vi "SSIM.vi"() -> ()   [LabVIEW 2014]
doc: "This example shows how to use the Structural Similarity Analysis tools in NI Vision. \n\nSSIM is a metric used to determine the Similarity of an Image with respect to a Reference Image. The Reference Image is assumed to be of perfect quality. SSIM uses a window based approach and uses the structural information to determine the similarity unlike the Mean Square Error which isolates the pixels from its neighbouring pixels.\n\nThere are two SSIM techniques. Fast and Normal SSIM. Fast SSIM uses faster approaches to calculate the mean and variance. Fast SSIM calculates mean by averaging pixel values in the local window whereas Normal SSIM uses a Gaussian weighting function."
uses:
  <vilib>/vision/NI_Vision_Development_Module.lvlib
panel:
  in  "Reference Image File Path":path
  in  "Window Size":i32=8 min=3 max=65
  out "MSE Map":T1(plugin-control)
  out "Mean Square Error":dbl
  in  "Test Image File Path":path
  out "Mean SSIM*":dbl
  in  "Fast/Normal":bool=TRUE
  out "SSIM Map":T1(plugin-control)
  out "Test Image":T1(plugin-control)
  out "Reference Image":T1(plugin-control)
  in  "Stop":bool
  # "Overview: Demonstrates how to compare two image using SSIM algorithm.\nRequirements: NI Vision Development Module\nInstructions:\n1. Run the VI\n2. Select different images using the Test Image File Path control\n3. Compare the SSIM similarity metric result to a simple mean square error computation."
  # "Comparison Results"
  # "SSIM Options"
  # "* In SSIM the value 1 indicates the images are similar, the value 0 indicates the images are dissimilar."
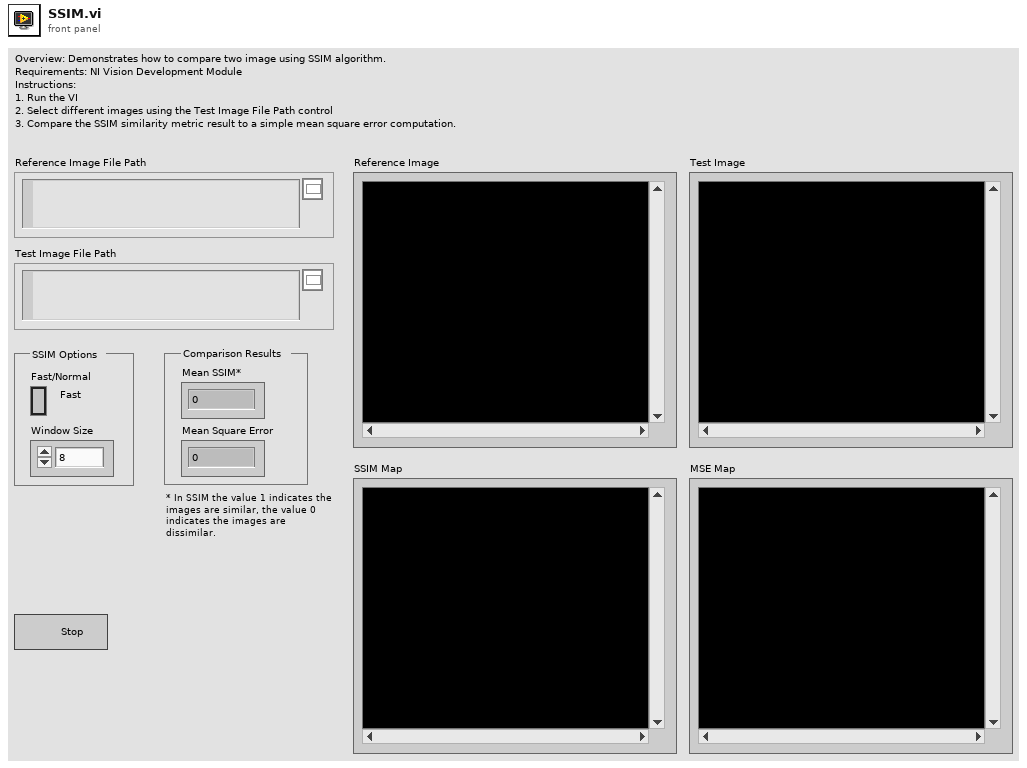
[diagram p1: front panel]
types:
  T1 = typedef "IMAQ Image.ctl" = refnum<image>
  T2 = typedef "Image Type" = u32
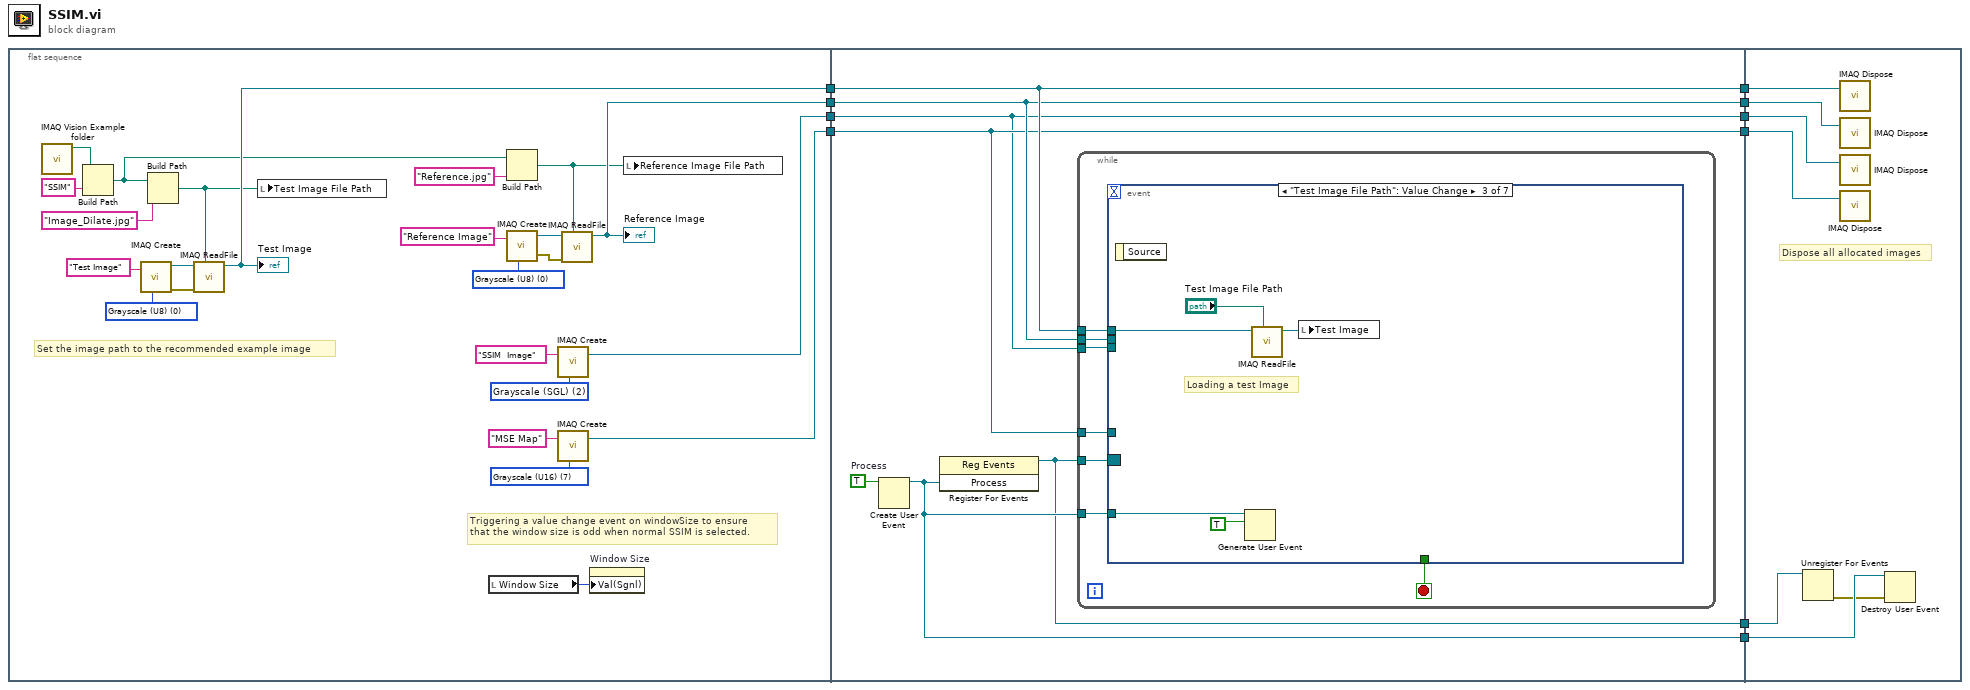
[diagram p0: block diagram]
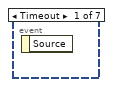
[diagram p2: hidden frame]
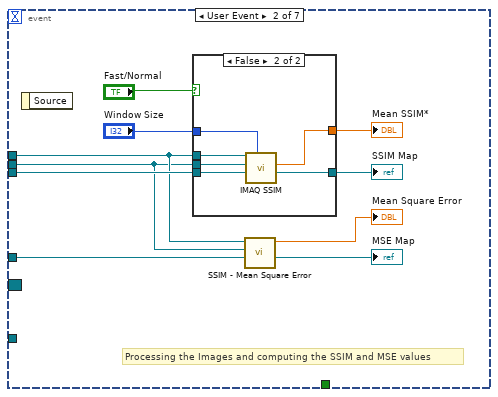
[diagram p3: hidden frame]
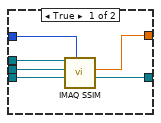
[diagram p4: hidden frame]
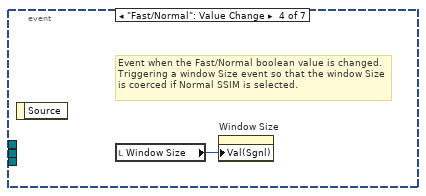
[diagram p5: hidden frame]
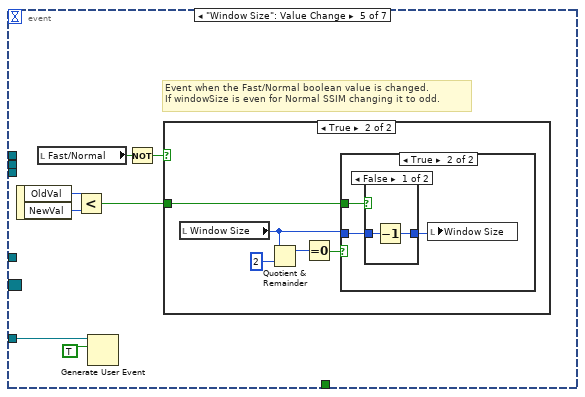
[diagram p6: hidden frame]
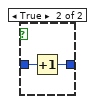
[diagram p9: hidden frame]
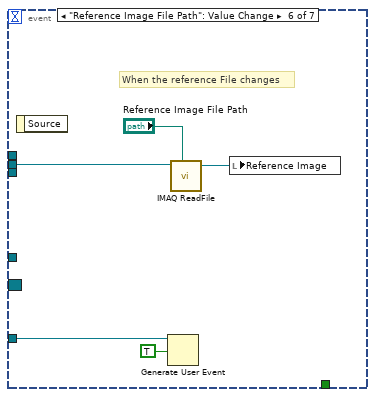
[diagram p10: hidden frame]
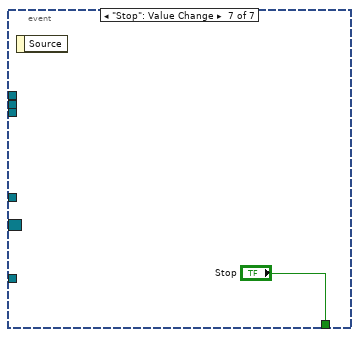
[diagram p11: hidden frame]
diagram:
  n1 = flat-sequence {
    tunnel: [w15] -> w10
    tunnel: [w14] -> w9
    tunnel: [w23] -> w8
    tunnel: [w20] -> w7
    tunnel: w10 -> [w41]
    tunnel: [w41] -> w6
    tunnel: w9 -> [w35]
    tunnel: [w35] -> w5
    tunnel: w8 -> [w40]
    tunnel: [w40] -> w4
    tunnel: w7 -> [w38]
    tunnel: [w38] -> w3
    tunnel: [w37] -> w2
    tunnel: [w36] -> w1
    tunnel: w6 -> [w108]
    tunnel: w5 -> [w104]
    tunnel: w4 -> [w102]
    tunnel: w3 -> [w107]
    tunnel: w2 -> [w105]
    tunnel: w1 -> [w106]
    frame #0 {
      w21 = T2 7 items=["Grayscale (U8)", "Grayscale (I16)", "Grayscale (SGL)", "Complex (CSG)", "RGB (U32)", "HSL (U32)", "RGB (U64)", "Grayscale (U16)"] ("Image Type")
      w25 = T2 2 items=["Grayscale (U8)", "Grayscale (I16)", "Grayscale (SGL)", "Complex (CSG)", "RGB (U32)", "HSL (U32)", "RGB (U64)"] ("Image Type")
      w31 = T2 0 items=["Grayscale (U8)", "Grayscale (I16)", "Grayscale (SGL)", "Complex (CSG)", "RGB (U32)", "HSL (U32)", "RGB (U64)"] ("Image Type")
      w32 = T2 0 items=["Grayscale (U8)", "Grayscale (I16)", "Grayscale (SGL)", "Complex (CSG)", "RGB (U32)", "HSL (U32)", "RGB (U64)"] ("Image Type")
      # "Triggering a value change event on windowSize to ensure \nthat the window size is odd when normal SSIM is selected."
      # "Set the image path to the recommended example image"
      n2 = call "IMAQ Vision Example folder.vi"() -> ("Example Image Path"=w27:path)  [unwired: 11 in]
      n3 = Build Path(base path=w27, name or relative path="SSIM") -> (appended path=w11:path)
      n4 = call "IMAQ Create"("Image Name"="Test Image", "Image Type"=w32) -> ("New Image"=w18:T1, "error out"=w17:errorcluster)  [unwired: 2 in, 1 out]
      n5 = Build Path(base path=w11, name or relative path="Image_Dilate.jpg") -> (appended path=w12:path)
      n6 = call "IMAQ ReadFile"("File Path"=w12, "error in (no error)"=w17, "Image"=w18) -> ("Image Out"=w15:T1)  [unwired: 2 in, 6 out]
      "Test Image" <- w15
      n7 = local write "Test Image File Path"(w12) -> ()
      n8 = local read "Window Size"() -> (w19:i32)
      n9 = Build Path(base path=w11, name or relative path="Reference.jpg") -> (appended path=w13:path)
      n10 = call "IMAQ Create"("Image Name"="Reference Image", "Image Type"=w31) -> ("New Image"=w30:T1, "error out"=w29:errorcluster)  [unwired: 2 in, 1 out]
      n11 = call "IMAQ Create"("Image Name"="SSIM  Image", "Image Type"=w25) -> ("New Image"=w14:T1)  [unwired: 2 in, 2 out]
      n12 = call "IMAQ Create"("Image Name"="MSE Map", "Image Type"=w21) -> ("New Image"=w20:T1)  [unwired: 2 in, 2 out]
      n13 = call "IMAQ ReadFile"("File Path"=w13, "error in (no error)"=w29, "Image"=w30) -> ("Image Out"=w23:T1)  [unwired: 2 in, 6 out]
      "Reference Image" <- w23
      n14 = property on="Window Size" class="DigNum (strict)"("Val(Sgnl)"=w19) -> ()  [unwired: 2 in, 2 out]
      n15 = local write "Reference Image File Path"(w13) -> ()
    }
    frame #1 {
      w39 = TRUE  # Process
      n16 = Create User Event(user event datatype=w39) -> (user event=w37:refnum<user-event>)  [unwired: 1 in, 1 out]
      n17 = register-events(w37) -> (reference out=w36:refnum<event-registration>)  [unwired: 2 in, 1 out]
      n18 = while {
        tunnel: w41 -> [w48]
        tunnel: w35 -> [w47]
        tunnel: w40 -> [w46]
        tunnel: w38 -> [w45]
        tunnel: w37 -> [w44]
        tunnel: w36 -> [w42]
        stop <- w43 stop-if-true
        n19 = event shown="[2] \"Test Image File Path\": Value Change" {
          selector: w42 -> [_ _ _ _ _ _ _]
          dyn-events: _ -> [_ _ _ _ _ _ _]
          timeout: _ -> [_ _ _ _ _ _ _]
          tunnel: w48 -> [_ w53 w75 _ _ _ _]
          tunnel: w47 -> [_ w58 _ _ _ _ _]
          tunnel: w46 -> [_ w52 _ _ _ w100 _]
          tunnel: w45 -> [_ w51 _ _ _ _ _]
          tunnel: w44 -> [_ _ w73 _ w83 w96 _]
          tunnel: [_ _ _ _ _ _ "Stop"] -> w43
          event Timeout {
            n20 = event-data() -> ()  [unwired: 2 out]
          }
          event User Event {
            # "Processing the Images and computing the SSIM and MSE values"
            n21 = event-data() -> ()  [unwired: 2 out]
            n22 = case shown="False" "Fast/Normal" {
              tunnel: w53 -> [w61 w68]
              tunnel: w52 -> [w59 w67]
              tunnel: w58 -> [w64 w70]
              tunnel: [w63 w65] -> w56
              tunnel: [w62 w69] -> w57
              tunnel: "Window Size" -> [w60 w66]
              frame True {
                n23 = call-poly "IMAQ SSIM"("Window Size"=w60, "SSIM Image In"=w64, "Reference Image"=w59, "Test Image"=w61) -> ("SSIM Image Out"=w62:T1, "Mean SSIM"=w63:dbl)  [unwired: 1 in, 5 out]
              }
              frame False {
                n24 = call-poly "IMAQ SSIM"("Window Size"=w66, "SSIM Image In"=w70, "Reference Image"=w67, "Test Image"=w68) -> ("SSIM Image Out"=w69:T1, "Mean SSIM"=w65:dbl)  [unwired: 1 in, 5 out]
              }
            }
            "SSIM Map" <- w57
            "Mean SSIM*" <- w56
            n25 = call "SSIM - Mean Square Error.vi"("MSE Map"=w51, "Reference Image"=w52, "Test Image"=w53) -> ("MSE Map Out"=→"MSE Map":T1, "Mean Square Error"=→"Mean Square Error":dbl)  [unwired: 1 in, 6 out]
          }
          event "Test Image File Path": Value Change {
            # "Loading a test Image"
            n26 = event-data() -> ()  [unwired: 2 out]
            n27 = Generate User Event(user event=w73, event data cluster=TRUE ("event data")) -> ()  [unwired: 2 in, 2 out]
            n28 = call "IMAQ ReadFile"("File Path"="Test Image File Path", "Image"=w75) -> ("Image Out"=w72:T1)  [unwired: 3 in, 6 out]
            n29 = local write "Test Image"(w72) -> ()
          }
          event "Fast/Normal": Value Change {
            # "Event when the Fast/Normal boolean value is changed.\nTriggering a window Size event so that the window Size is coerced if Normal SSIM is selected."
            n30 = event-data() -> ()  [unwired: 2 out]
            n31 = local read "Window Size"() -> (w76:i32)
            n32 = property on="Window Size" class="DigNum (strict)"("Val(Sgnl)"=w76) -> ()  [unwired: 2 in, 2 out]
          }
          event "Window Size": Value Change {
            # "Event when the Fast/Normal boolean value is changed.\nIf windowSize is even for Normal SSIM changing it to odd."
            n33 = event-data() -> ("OldVal"=w79:i32, "NewVal"=w78:i32)  [unwired: 1 out]
            n34 = local read "Fast/Normal"() -> (w82:bool)
            n35 = Less?(x=w79, y=w78) -> (x < y?=w77:bool)
            n36 = Generate User Event(user event=w83, event data cluster=TRUE ("event data")) -> ()  [unwired: 2 in, 2 out]
            n37 = Not(x=w82) -> (.not. x?=w80:bool)
            n38 = case shown="True" w80 {
              tunnel: w77 -> [_ w85]
              frame False {
              }
              frame True {
                n39 = local read "Window Size"() -> (w86:i32)
                n40 = Quotient & Remainder(x=w86, y=2) -> (x-y*floor(x/y)=w84:i32)  [unwired: 1 out]
                n41 = Equal To 0?(x=w84) -> (x = 0?=w87:bool)
                n42 = case shown="True" w87 {
                  tunnel: w86 -> [_ w90]
                  tunnel: w85 -> [_ w91]
                  frame False {
                  }
                  frame True {
                    n43 = case shown="False" w91 {
                      tunnel: w90 -> [w92 w94]
                      tunnel: [w93 w95] -> w89
                      frame False {
                        n44 = Decrement(x=w92) -> (x-1=w93:i32)
                      }
                      frame True {
                        n45 = Increment(x=w94) -> (x+1=w95:i32)
                      }
                    }
                    n46 = local write "Window Size"(w89) -> ()
                  }
                }
              }
            }
          }
          event "Reference Image File Path": Value Change {
            # "When the reference File changes"
            n47 = event-data() -> ()  [unwired: 2 out]
            n48 = Generate User Event(user event=w96, event data cluster=TRUE ("event data")) -> ()  [unwired: 2 in, 2 out]
            n49 = call "IMAQ ReadFile"("File Path"="Reference Image File Path", "Image"=w100) -> ("Image Out"=w98:T1)  [unwired: 3 in, 6 out]
            n50 = local write "Reference Image"(w98) -> ()
          }
          event "Stop": Value Change {
            n51 = event-data() -> ()  [unwired: 2 out]
          }
        }
      }
    }
    frame #2 {
      # "Dispose all allocated images"
      n52 = Unregister For Events(event registration refnum=w106) -> (error out=w103:errorcluster)  [unwired: 1 in]
      n53 = call "IMAQ Dispose"("Image"=w108) -> ()  [unwired: 2 in, 4 out]
      n54 = call "IMAQ Dispose"("Image"=w102) -> ()  [unwired: 2 in, 4 out]
      n55 = call "IMAQ Dispose"("Image"=w104) -> ()  [unwired: 2 in, 4 out]
      n56 = call "IMAQ Dispose"("Image"=w107) -> ()  [unwired: 2 in, 4 out]
      n57 = Destroy User Event(user event=w105, error in=w103) -> ()  [unwired: 1 out]
    }
  }
